vi "Печать.vi"() -> ()   [LabVIEW 2021]
panel:
  in  "Выкл":bool
  out "Сообщение":string
  in  "Бумага":dbl
  in  "Черннила":u8(slide) scale=0.0..100.0
  in  "Меню":T1
  out "Slide":u8(slide) scale=0.0..100.0
  in  "Вкл":bool
  out "Enum":T2
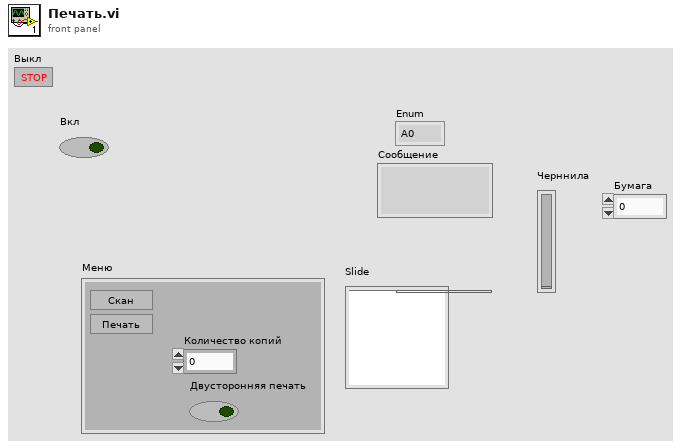
[diagram p1: front panel]
types:
  T1 = typedef "Меню печати.ctl" = cluster{"Скан":bool, "Количество копий":dbl, "Двусторонняя печать":bool, "Печать\n":bool}
  T2 = typedef "Печать.ctl" = enum16{"А0", "Анализ ошибок", "Выбор пользователя", "Печать", "Скан"}
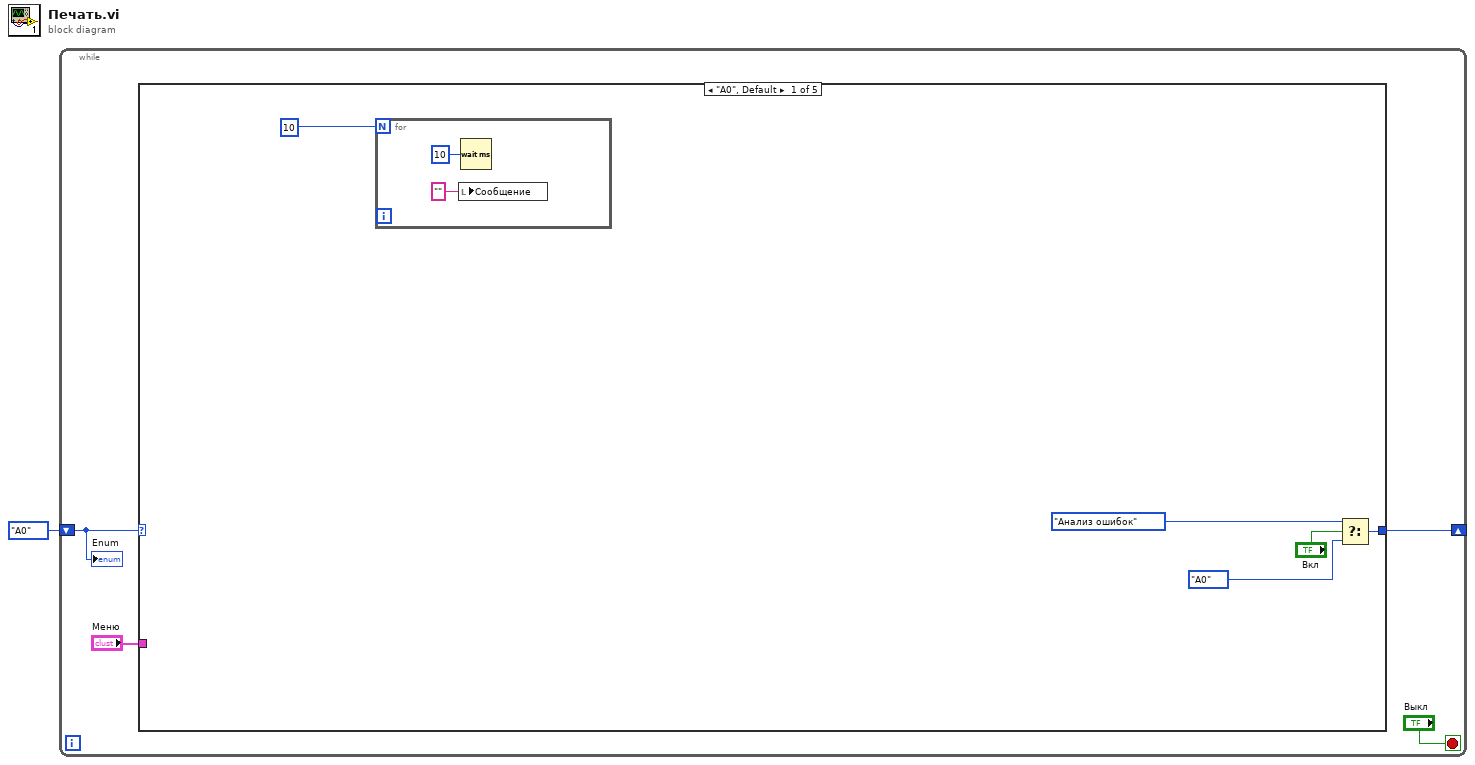
[diagram p0: block diagram]
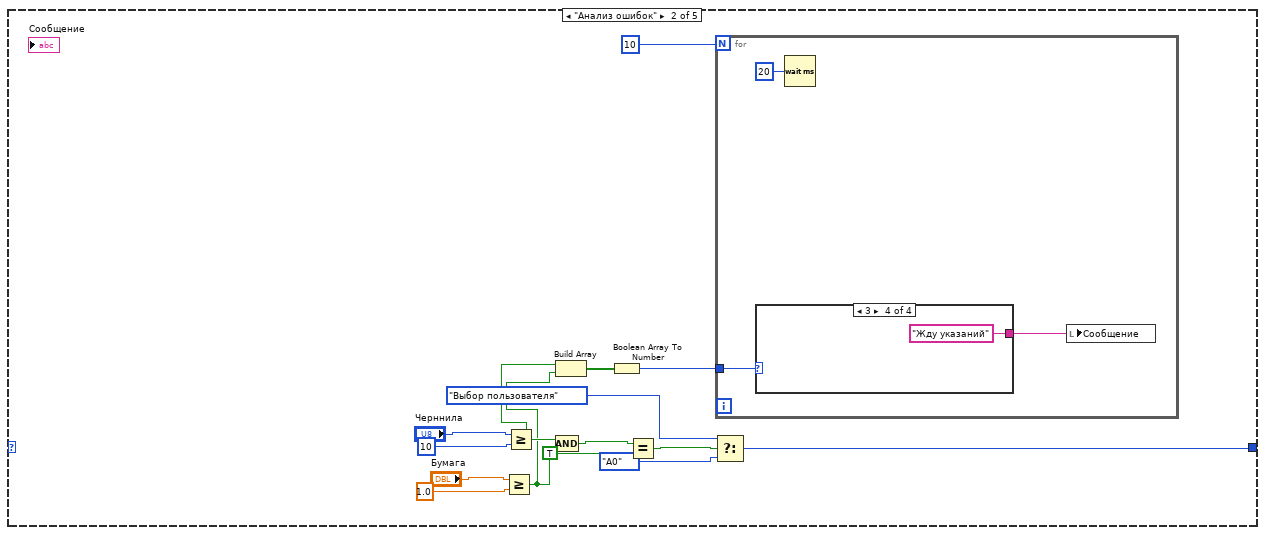
[diagram p2: hidden frame]
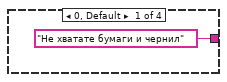
[diagram p3: hidden frame]
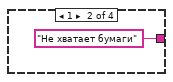
[diagram p4: hidden frame]
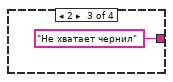
[diagram p5: hidden frame]
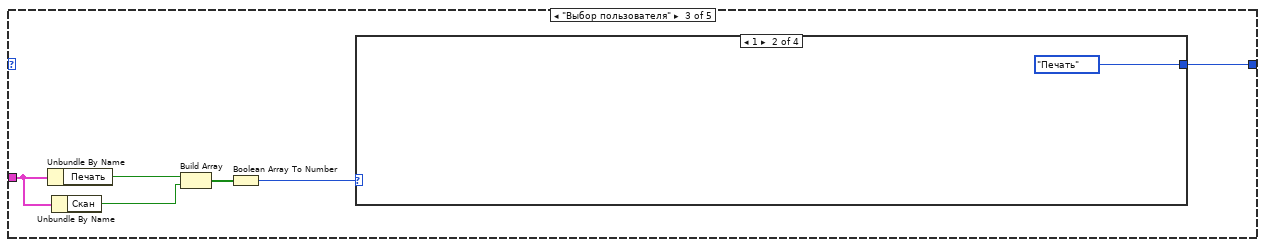
[diagram p6: hidden frame]
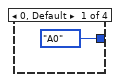
[diagram p7: hidden frame]
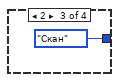
[diagram p8: hidden frame]
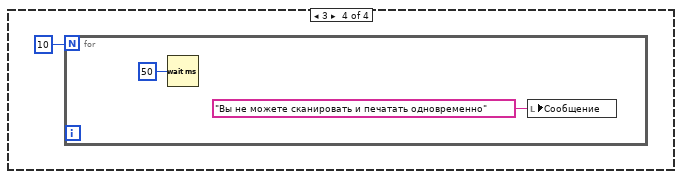
[diagram p9: hidden frame]
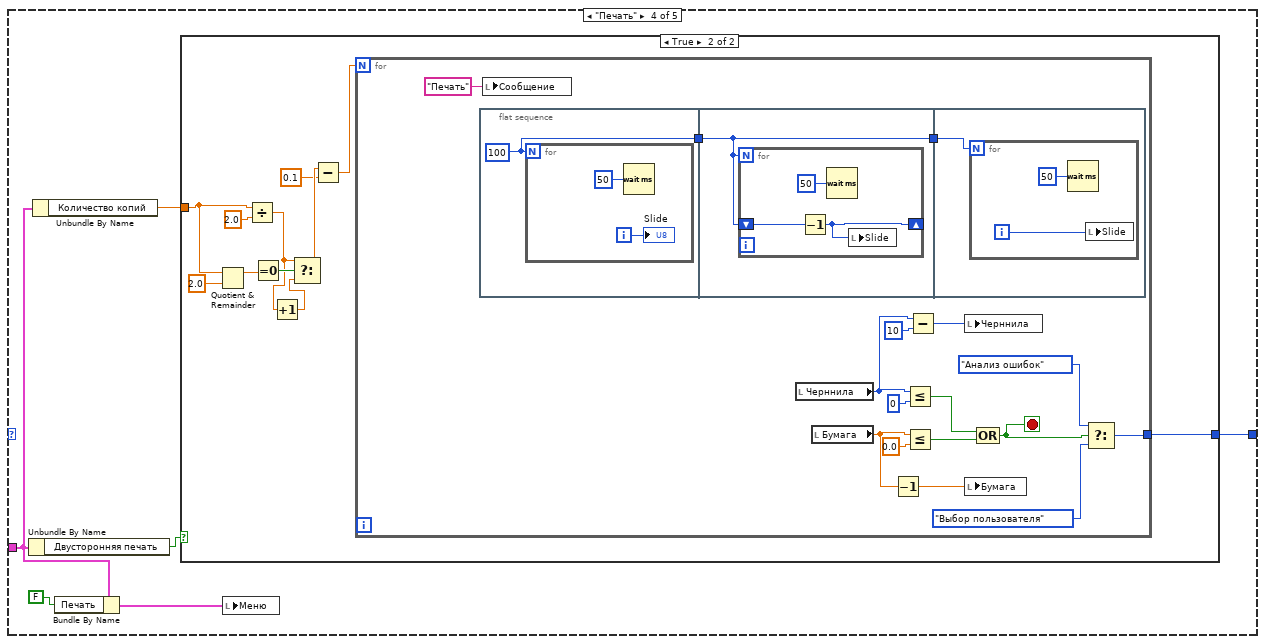
[diagram p10: hidden frame]
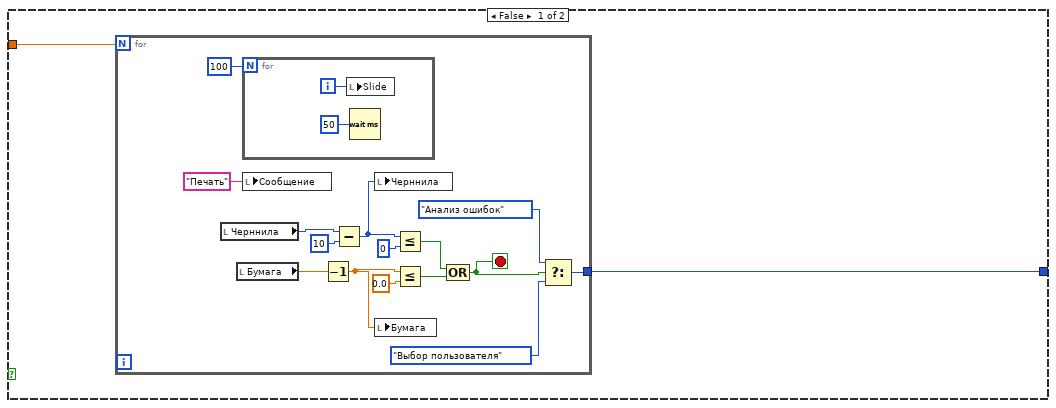
[diagram p11: hidden frame]
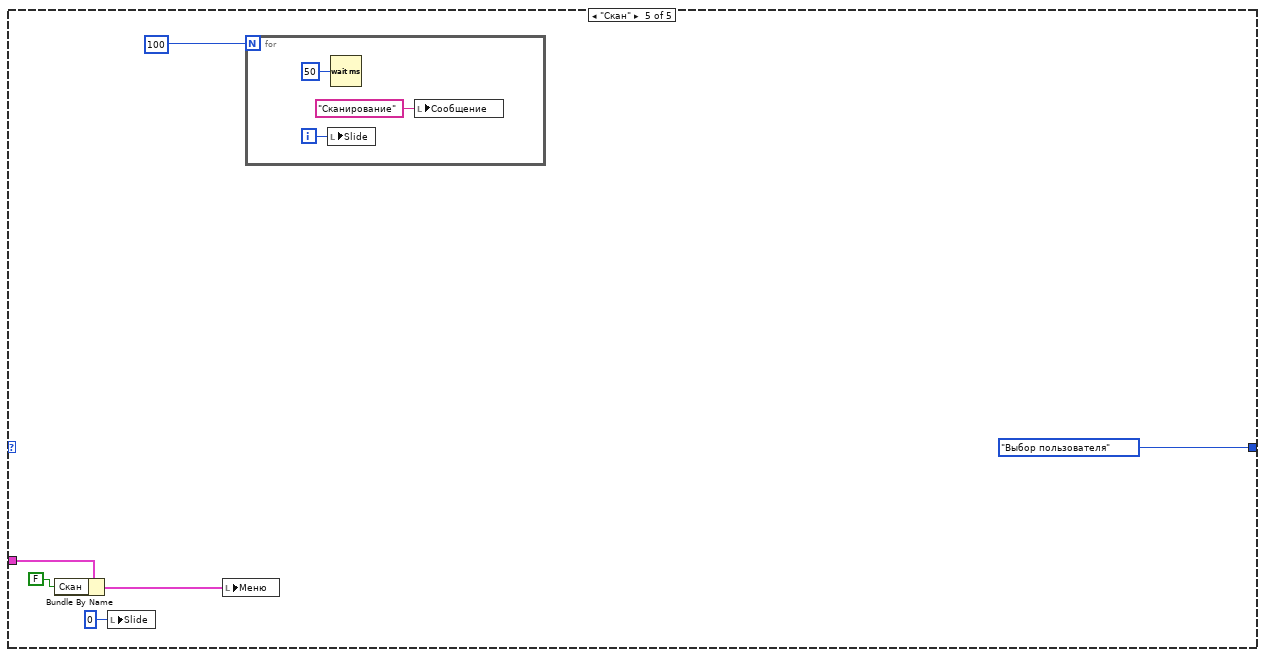
[diagram p12: hidden frame]
diagram:
  n1 = while {
    shift-right: [w5] -> _
    shift-left: Печать."А0" ("Enum") -> [w2]
    stop <- "Выкл" stop-if-true
    n2 = case shown="\"А0\", Default" w2 {
      tunnel: [w7 w17 w38 w47 Печать."Выбор пользователя" ("Enum")] -> w5
      tunnel: "Меню" -> [_ _ w37 w49 w110]
      frame "А0", Default {
        n3 = for {
          N: 10 -> [_]
          n4 = local write "Сообщение"("" ("Сообщение")) -> ()
          n5 = Wait (ms)(milliseconds to wait=u32 10) -> ()  [unwired: 1 out]
        }
        n6 = Select(t=Печать."Анализ ошибок" ("Enum"), s="Вкл", f=Печать."А0" ("Enum")) -> (s? t:f=w7:T2)
      }
      frame "Анализ ошибок" {
        n7 = Greater Or Equal?(x="Бумага", y=1.0) -> (x >= y?=w19:bool)
        n8 = Greater Or Equal?(x="Черннила", y=u8 10) -> (x >= y?=w20:bool)
        n9 = Build Array(w20, w19) -> (w21:bool[])
        n10 = Compound Arithmetic op=AND(w20, w19) -> (w16:bool)
        n11 = Boolean Array To Number(Boolean array=w21) -> (number=w18:u32)
        n12 = Equal?(x=w16, y=TRUE) -> (x = y?=w14:bool)
        n13 = Select(t=Печать."Выбор пользователя" ("Enum"), s=w14, f=Печать."А0" ("Enum")) -> (s? t:f=w17:T2)
        n14 = for {
          N: 10 -> [_]
          tunnel: w18 -> [w30]
          n15 = case shown="3" w30 {
            tunnel: ["Не хватате бумаги и чернил" "Не хватает бумаги" "Не хватает чернил" "Жду указаний"] -> w28
            frame 0, Default {
            }
            frame 1 {
            }
            frame 2 {
            }
            frame 3 {
            }
          }
          n16 = Wait (ms)(milliseconds to wait=u32 20) -> ()  [unwired: 1 out]
          n17 = local write "Сообщение"(w28) -> ()
        }
      }
      frame "Выбор пользователя" {
        n18 = Unbundle By Name(w37) -> ("Печать"=w36:bool)
        n19 = Unbundle By Name(w37) -> ("Скан"=w35:bool)
        n20 = Build Array(w36, w35) -> (w40:bool[])
        n21 = Boolean Array To Number(Boolean array=w40) -> (number=w39:u32)
        n22 = case shown="1" w39 {
          tunnel: [Печать."А0" ("Enum") Печать."Печать" ("Enum") Печать."Скан" ("Enum") _] -> w38
          frame 0, Default {
          }
          frame 1 {
          }
          frame 2 {
          }
          frame 3 {
            n23 = for {
              N: 10 -> [_]
              n24 = Wait (ms)(milliseconds to wait=u32 50) -> ()  [unwired: 1 out]
              n25 = local write "Сообщение"("Вы не можете сканировать и печатать одновременно" ("Сообщение")) -> ()
            }
          }
        }
      }
      frame "Печать" {
        n26 = Unbundle By Name(w49) -> ("Двусторонняя печать"=w51:bool)
        n27 = Unbundle By Name(w49) -> ("Количество копий"=w52:dbl)
        n28 = Bundle By Name(cluster=w49, "Печать"=FALSE) -> (w50:T1)
        n29 = case shown="True" w51 {
          tunnel: w52 -> [w54 w80]
          tunnel: [w53 w81] -> w47
          frame False {
            n30 = for {
              N: w54 -> [_]
              tunnel: [w57] -> w53
              stop <- w59 stop-if-true
              n31 = local read "Черннила"() -> (w67:u8)
              n32 = local read "Бумага"() -> (w68:dbl)
              n33 = for {
                N: 100 -> [_]
                i -> [w70]
                n34 = local write "Slide"(w70) -> ()
                n35 = Wait (ms)(milliseconds to wait=u32 50) -> ()  [unwired: 1 out]
              }
              n36 = local write "Сообщение"("Печать" ("Сообщение")) -> ()
              n37 = Decrement(x=w68) -> (x-1=w56:dbl)
              n38 = Subtract(x=w67, y=u8 10) -> (x-y=w55:u8)
              n39 = local write "Черннила"(w55) -> ()
              n40 = local write "Бумага"(w56) -> ()
              n41 = Less Or Equal?(x=w55, y=u8 0) -> (x <= y?=w66:bool)
              n42 = Less Or Equal?(x=w56, y=0.0) -> (x <= y?=w65:bool)
              n43 = Compound Arithmetic op=OR(w66, w65) -> (w59:bool)
              n44 = Select(t=Печать."Анализ ошибок" ("Enum"), s=w59, f=Печать."Выбор пользователя" ("Enum")) -> (s? t:f=w57:T2)
            }
          }
          frame True {
            n45 = Quotient & Remainder(x=w80, y=2.0) -> (x-y*floor(x/y)=w78:dbl)  [unwired: 1 out]
            n46 = Divide(x=w80, y=2.0) -> (x/y=w76:dbl)
            n47 = Equal To 0?(x=w78) -> (x = 0?=w77:bool)
            n48 = Increment(x=w76) -> (x+1=w75:dbl)
            n49 = Select(t=w76, s=w77, f=w75) -> (s? t:f=w73:dbl)
            n50 = Subtract(x=w73, y=0.1) -> (x-y=w74:dbl)
            n51 = for {
              N: w74 -> [_]
              tunnel: [w85] -> w81
              stop <- w87 stop-if-true
              n52 = flat-sequence {
                tunnel: [w99] -> w84
                tunnel: w84 -> [w102]
                tunnel: [w102] -> w83
                tunnel: w83 -> [w106]
                frame #0 {
                  w99 = 100
                  n53 = for {
                    N: w99 -> [_]
                    i -> [w100]
                    n54 = Wait (ms)(milliseconds to wait=u32 50) -> ()  [unwired: 1 out]
                    "Slide" <- w100
                  }
                }
                frame #1 {
                  n55 = for {
                    N: w102 -> [_]
                    shift-right: [w103] -> _
                    shift-left: w102 -> [w104]
                    n56 = Decrement(x=w104) -> (x-1=w103:i32)
                    n57 = Wait (ms)(milliseconds to wait=u32 50) -> ()  [unwired: 1 out]
                    n58 = local write "Slide"(w103) -> ()
                  }
                }
                frame #2 {
                  n59 = for {
                    N: w106 -> [_]
                    i -> [w107]
                    n60 = Wait (ms)(milliseconds to wait=u32 50) -> ()  [unwired: 1 out]
                    n61 = local write "Slide"(w107) -> ()
                  }
                }
              }
              n62 = local write "Сообщение"("Печать" ("Сообщение")) -> ()
              n63 = local read "Черннила"() -> (w92:u8)
              n64 = local read "Бумага"() -> (w94:dbl)
              n65 = Decrement(x=w94) -> (x-1=w98:dbl)
              n66 = Less Or Equal?(x=w92, y=u8 0) -> (x <= y?=w90:bool)
              n67 = Less Or Equal?(x=w94, y=0.0) -> (x <= y?=w89:bool)
              n68 = Subtract(x=w92, y=u8 10) -> (x-y=w97:u8)
              n69 = local write "Черннила"(w97) -> ()
              n70 = local write "Бумага"(w98) -> ()
              n71 = Compound Arithmetic op=OR(w90, w89) -> (w87:bool)
              n72 = Select(t=Печать."Анализ ошибок" ("Enum"), s=w87, f=Печать."Выбор пользователя" ("Enum")) -> (s? t:f=w85:T2)
            }
          }
        }
        n73 = local write "Меню"(w50) -> ()
      }
      frame "Скан" {
        n74 = Bundle By Name(cluster=w110, "Скан"=FALSE ("Печать")) -> (w111:T1)
        n75 = local write "Slide"(u8 0 ("Slide")) -> ()
        n76 = local write "Меню"(w111) -> ()
        n77 = for {
          N: 100 -> [_]
          i -> [w116]
          n78 = local write "Slide"(w116) -> ()
          n79 = Wait (ms)(milliseconds to wait=u32 50) -> ()  [unwired: 1 out]
          n80 = local write "Сообщение"("Сканирование" ("Сообщение")) -> ()
        }
      }
    }
    "Enum" <- w2
  }
